vi "fuzzy_ctrl.vi"() -> ()   [LabVIEW 2022 SP3]
uses:
  <vilib>/addons/Fuzzy Logic/FL Fuzzy Controller (MISO).vi
  <vilib>/addons/Fuzzy Logic/NI_Fuzzy_Logic_API.lvlib
panel:
  in  "Mode":bool
  in  "ym":dbl(slide) caption="Measurement" scale=-10.0..10.0
  in  "set_point":dbl(knob) caption="SP" scale=-10.0..10.0
  out "delta_error":dbl(knob) caption="Error Rate" scale=-10.0..10.0
  out "array of clusters":cluster{"Color":u32, "String":string}[](array[cluster]) caption="Rules"
  out "error out":errorcluster
  out "out":dbl(knob) caption="Output" scale=-10.0..10.0
  in  "Stop Button":bool
  # "SIM"
  # "RPI"
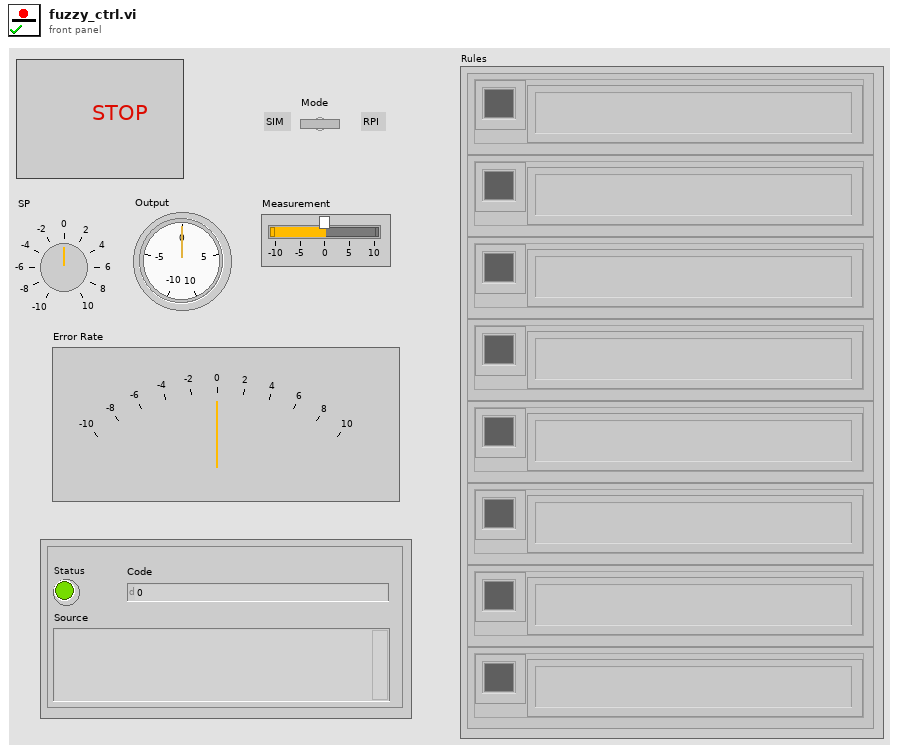
[diagram p1: front panel]
types:
  T1 = typedef "NI_Fuzzy_Logic_API.lvlib/FL System.ctl" = cluster{"input variables":T2[], "output variables":T2[], "rules":T5[], "defuzzification method":T11, "description":string, "user MF interpolating polynomials":T12[]}
  T2 = typedef "NI_Fuzzy_Logic_API.lvlib/FL Variable.ctl" = cluster{"name":string, "range":dbl[], "MFs":T3[]}
  T3 = typedef "NI_Fuzzy_Logic_API.lvlib/FL Membership Function.ctl" = cluster{"name":string, "shape":T4, "points":dbl[], "color":u32, "user-defined shape index":i32}
  T4 = typedef "NI_Fuzzy_Logic_API.lvlib/FL Membership Function Shape.ctl" = u16
  T5 = typedef "NI_Fuzzy_Logic_API.lvlib/FL Rule.ctl" = cluster{"antecedents":T6[], "antecedent connective":T8, "consequents":T9[], "consequent implication":T10, "degree of support":dbl}
  T6 = typedef "NI_Fuzzy_Logic_API.lvlib/FL Antecedent.ctl" = cluster{"Var Index":i32, "MF Index":i32, "Cond":T7}
  T7 = typedef "NI_Fuzzy_Logic_API.lvlib/FL Modifier.ctl" = u16
  T8 = typedef "NI_Fuzzy_Logic_API.lvlib/FL Antecedent Connective.ctl" = u16
  T9 = typedef "NI_Fuzzy_Logic_API.lvlib/FL Consequent.ctl" = cluster{"Var Index":i32, "MF Index":i32, "Cond":T7}
  T10 = typedef "NI_Fuzzy_Logic_API.lvlib/FL Consequent Implication.ctl" = u16
  T11 = typedef "NI_Fuzzy_Logic_API.lvlib/FL Defuzzification.ctl" = u16
  T12 = typedef "NI_Fuzzy_Logic_API.lvlib/FL Interpolating polynomials.ctl" = cluster{"X":dbl[], "Y":dbl[], "Y(x) coeff":dbl[][], "X(y) coeff":dbl[][], "Area(y) coeff":dbl[][], "coa_x(y) coeff":dbl[][]}
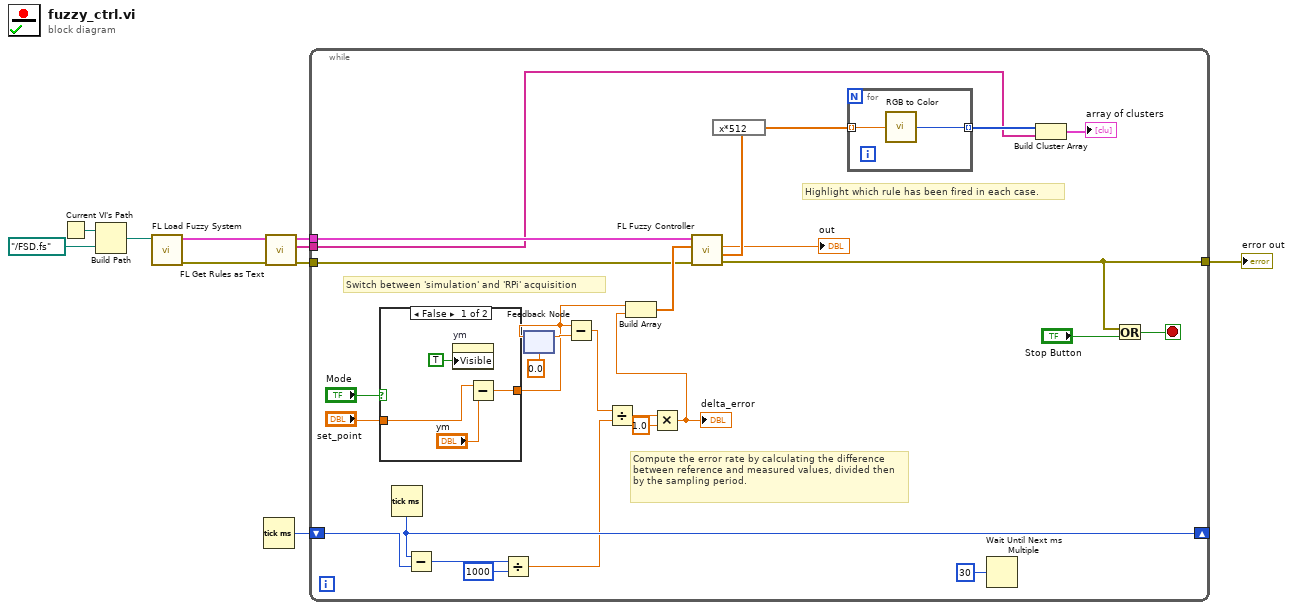
[diagram p0: block diagram]
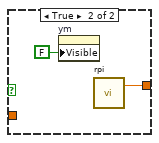
[diagram p2: hidden frame]
diagram:
  n1 = Current VI's Path() -> (path=w9:path)
  n2 = Build Path(base path=w9, name or relative path=path "../FSD.fs") -> (appended path=w8:path)
  n3 = call <vilib>:"FL Load Fuzzy System.vi"("file path"=w8) -> ("error out"=w5:errorcluster, "fuzzy system out"=w6:T1)  [unwired: 9 in]
  n4 = Tick Count (ms)() -> (millisecond timer value=w1:u32)
  n5 = call <vilib>:"FL Get Rules as Text.vi"("error in (no error)"=w5, "fuzzy system in"=w6) -> ("error out"=w3:errorcluster, "rules as text"=w2:string[], "fuzzy system out"=w4:T1)  [unwired: 7 in]
  n6 = while {
    tunnel: w4 -> [w36]
    tunnel: [w32] -> w7
    tunnel: w3 -> [w31]
    tunnel: w2 -> [w26]
    shift-right: [w13] -> _
    shift-left: w1 -> [w12]
    stop <- w34 stop-if-true
    # "Highlight which rule has been fired in each case."
    # "Switch between 'simulation' and 'RPi' acquisition"
    # "Compute the error rate by calculating the difference between reference and measured values, divided then by the sampling period."
    n7 = case shown="False" "Mode" {
      tunnel: [w41 w43] -> w16
      tunnel: "set_point" -> [w40 _]
      frame False {
        n8 = property on="ym" class="Slide (strict)"("Visible"=TRUE) -> ()  [unwired: 2 in, 2 out]
        n9 = Subtract(x=w40, y="ym") -> (x-y=w41:dbl)
      }
      frame True {
        n10 = property on="ym" class="Slide (strict)"("Visible"=FALSE) -> ()  [unwired: 2 in, 2 out]
        n11 = call "rpi.vi"() -> ("measured_output"=w43:dbl)  [unwired: 3 in]
      }
    }
    n12 = Tick Count (ms)() -> (millisecond timer value=w13:u32)
    n13 = Subtract(x=w13, y=w12) -> (x-y=w22:u32)
    n14 = Divide(x=w22, y=u32 1000) -> (x/y=w11:dbl)
    n15 = feedback-in #1(w16) -> ()
    n16 = feedback #1(0.0 ("error")) -> (w24:dbl)
    n17 = Subtract(x=w16, y=w24) -> (x-y=w23:dbl)
    n18 = Divide(x=w23, y=w11) -> (x/y=w20:dbl)
    n19 = Multiply(x=w20, y=1.0) -> (x*y=w18:dbl)
    "delta_error" <- w18
    n20 = Build Array(w16, w18) -> (w37:dbl[])
    n21 = call-poly <vilib>:"FL Fuzzy Controller.vi"("error in (no error)"=w31, "input values"=w37, "fuzzy system in"=w36) -> ("error out"=w32:errorcluster, "rule weights"=w29:dbl[], "output value"=→"out":dbl)  [unwired: 4 in, 2 out]
    n22 = expression code="x*512"(w29) -> (w30:dbl[])
    n23 = for {
      tunnel: [w45] -> w27 mode=indexing
      tunnel: w30 -> [w44] mode=indexing
      n24 = call <vilib>:"RGB to Color.vi"("G"=w44) -> ("Color"=w45:u32)  [unwired: 2 in]
    }
    n25 = Wait Until Next ms Multiple(millisecond multiple=u32 30) -> ()  [unwired: 1 out]
    n26 = Build Cluster Array(w27, w26) -> (→"array of clusters":cluster{"Color":u32, string}[])
    n27 = Or(x=w32, y="Stop Button") -> (x .or. y?=w34:bool)
  }
  "error out" <- w7
